vi "Create 7z config.vi"(8 "error in (no error)":errorcluster, 11 "PostBuildSupport in":refnum<class "PostBuildSupport.lvclass">) -> (0 "error out":errorcluster, 2 "resulting string":string, 3 "PostBuildSupport out":refnum<class "PostBuildSupport.lvclass">)   [LabVIEW 2019, in "PostBuildSupport.lvclass"]
uses:
  PostBuildSupport.lvclass
  PostBuildSupport.lvclass/PostBuildSupport.ctl
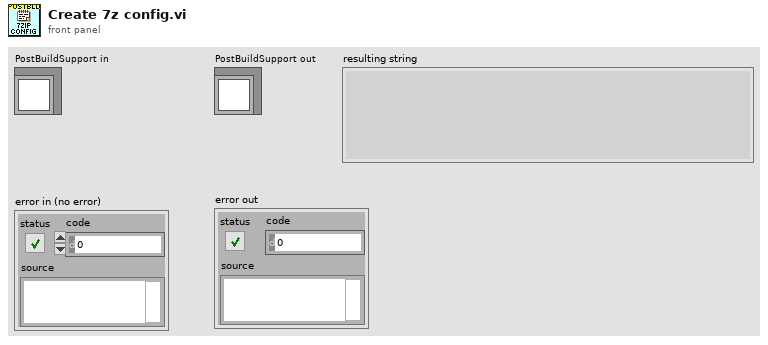
[diagram p1: front panel]
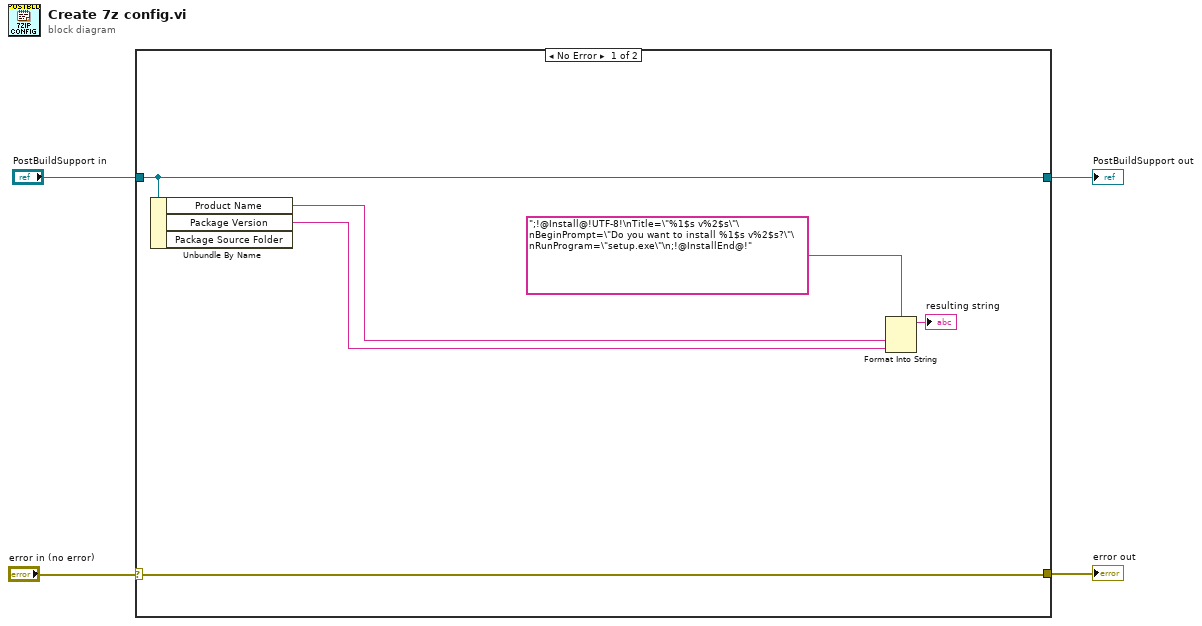
[diagram p0: block diagram]
diagram:
  n1 = case shown="No Error" "error in (no error)" {
    selector: "error in (no error)" -> [w5 w11]
    tunnel: [w5 w11] -> w4
    tunnel: "PostBuildSupport in" -> [w10 w12]
    tunnel: [w10 w12] -> w2
    frame No Error {
      n2 = Unbundle By Name(w10) -> ("Product Name"=w8:string, "Package Version"=w6:string)  [unwired: 1 out]
      n3 = Format Into String(format string=";!@Install@!UTF-8!\nTitle=\"%1$s v%2$s\"\nBeginPrompt=\"Do you want to install %1$s v%2$s?\"\nRunProgram=\"setup.exe\"\n;!@InstallEnd@!" ("Name of target (My Computer)"), w8, w6) -> (resulting string=→"resulting string":string)  [unwired: 2 in, 1 out]
    }
    frame Error {
    }
  }
  "error out" <- w4
  "PostBuildSupport out" <- w2
